vi "AlliGator Optimal Lifetime Guess.vi"(8 "error in (no error)":errorcluster, 9 "Delta tau Array":dbl[](array[numeric]), 11 "Guessed tau Array":dbl[](array[numeric])) -> (0 "error out":errorcluster, 1 "-t*_0/s Array":dbl[](array[numeric]))   [LabVIEW 2021, in "AlliGator IRF.lvlib"]
uses:
  AlliGator IRF.lvlib
  <vilib>/Analysis/NI_AALPro.lvlib
panel:
  out "Waveform Graph":dbl[](graph)
  # "see the License on the block diagram (Ctrl+E or Window:Show Block Diagram)"
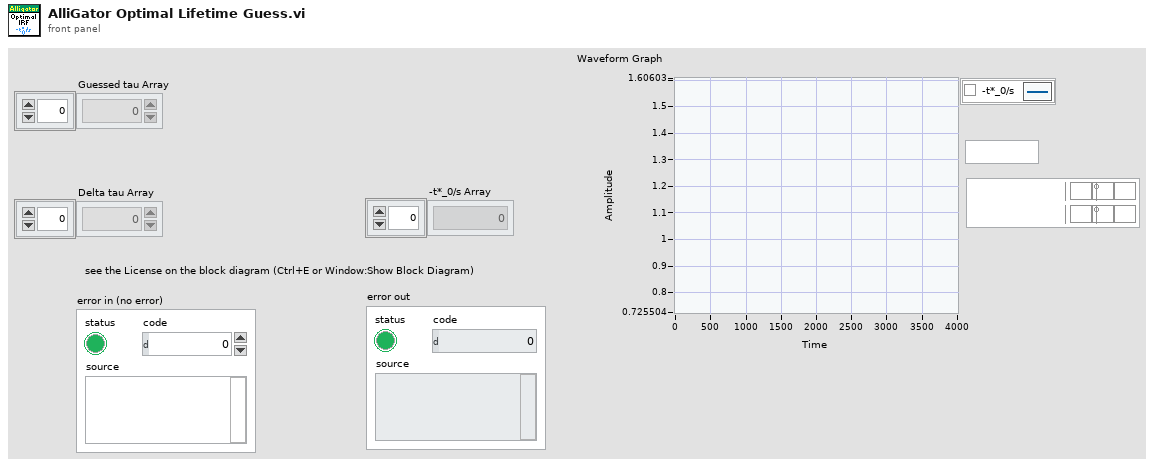
[diagram p1: front panel]
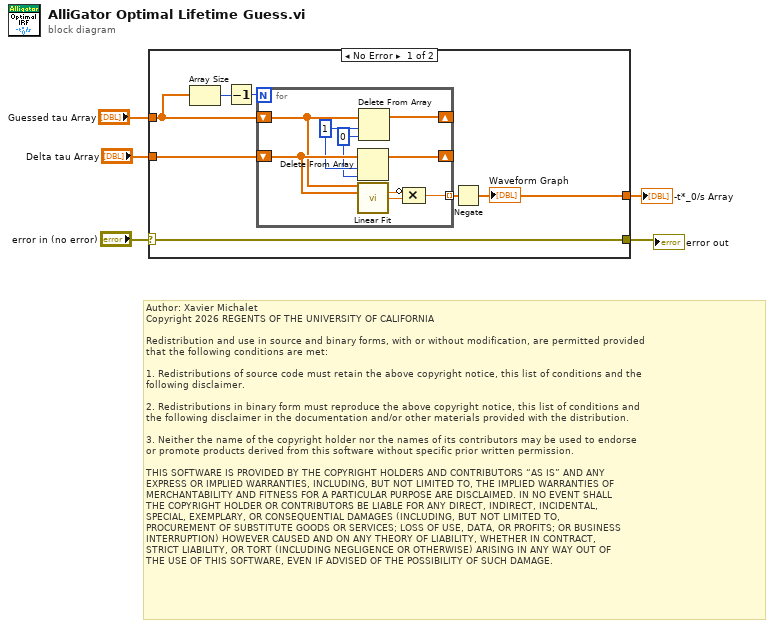
[diagram p0: block diagram]
diagram:
  # "Author: Xavier Michalet\nCopyright 2026 REGENTS OF THE UNIVERSITY OF CALIFORNIA\n\nRedistribution and use in source and binary forms, with or without modification, are permitted provided\nthat the following conditions are met:\n\n1. Redistributions of source code must retain the above copyright notice, this list of conditions and the\nfollowing disclaimer.\n\n2. Redistributions in binary form must reproduce the above copyright notice, this list of conditions and\nthe following disclaimer in the documentation and/or other materials provided with the distribution.\n\n3. Neither the name of the copyright holder nor the names of its contributors may be used to endorse \nor promote products derived from this software without specific prior written permission.\n\nTHIS SOFTWARE IS PROVIDED BY THE COPYRIGHT HOLDERS AND CONTRIBUTORS “AS IS” AND ANY \nEXPRESS OR IMPLIED WARRANTIES, INCLUDING, BUT NOT LIMITED TO, THE IMPLIED WARRANTIES OF\nMERCHANTABILITY AND FITNESS FOR A PARTICULAR PURPOSE ARE DISCLAIMED. IN NO EVENT SHALL\nTHE COPYRIGHT HOLDER OR CONTRIBUTORS BE LIABLE FOR ANY DIRECT, INDIRECT, INCIDENTAL, \nSPECIAL, EXEMPLARY, OR CONSEQUENTIAL DAMAGES (INCLUDING, BUT NOT LIMITED TO, \nPROCUREMENT OF SUBSTITUTE GOODS OR SERVICES; LOSS OF USE, DATA, OR PROFITS; OR BUSINESS\nINTERRUPTION) HOWEVER CAUSED AND ON ANY THEORY OF LIABILITY, WHETHER IN CONTRACT, \nSTRICT LIABILITY, OR TORT (INCLUDING NEGLIGENCE OR OTHERWISE) ARISING IN ANY WAY OUT OF\nTHE USE OF THIS SOFTWARE, EVEN IF ADVISED OF THE POSSIBILITY OF SUCH DAMAGE."
  n1 = case shown="No Error" "error in (no error)" {
    selector: "error in (no error)" -> [w10 w22]
    tunnel: "Delta tau Array" -> [w9 _]
    tunnel: "Guessed tau Array" -> [w8 _]
    tunnel: [w10 w22] -> w2
    tunnel: [w6 _] -> w1
    frame No Error {
      n2 = Array Size(array=w8) -> (size(s)=w12:i32)
      n3 = Decrement(x=w12) -> (x-1=w11:i32)
      n4 = for {
        N: w11 -> [_]
        shift-right: [w15] -> _
        shift-left: w9 -> [w21]
        shift-right: [w16] -> _
        shift-left: w8 -> [w20]
        tunnel: [w17] -> w7 mode=indexing
        w14 = 1 ("length")
        w13 = 0 ("index")
        n5 = Delete From Array(array=w21, length=w14, index=w13) -> (array with subset deleted=w15:dbl[])  [unwired: 1 out]
        n6 = call <vilib>:"Linear Fit.vi"("Y"=w20, "X"=w21) -> ("slope"=w19:dbl, "intercept"=w18:dbl)  [unwired: 9 in, 3 out]
        n7 = Delete From Array(array=w20, length=w14, index=w13) -> (array with subset deleted=w16:dbl[])  [unwired: 1 out]
        n8 = Compound Arithmetic op=MULTIPLY(invert w19, w18) -> (w17:dbl)
      }
      n9 = Negate(x=w7) -> (-x=w6:dbl[])
      "Waveform Graph" <- w6
    }
    frame Error {
    }
  }
  "error out" <- w2
  "-t*_0/s Array" <- w1
